vi "WriteWfmToDAQ.vi"(0 "clock settings":T3={"sample mode"=10178, "samples per channel"=1000, "rate"=1000.0} {"sample mode" items=["Finite Samples"=10178, "Continuous Samples"=10123, "Hardware Timed Single Point"=12522]}, 5 "channel settings":T2={"max value"=5.0, "min value"=-5.0, "physical channels"="Dev1/ai2", "input terminal configuration"=-1, "units"=10348} {"input terminal configuration" items=["Default"=-1, "RSE"=10083, "NRSE"=10078, "Differential"=10106, "Pseudodifferential"=12529]; "units" items=["Volts"=10348, "From Custom Scale"=10065]}, 9 "FuncGen settings":T1={"signal type"=enum."Sine Wave", "amplitude"=1.0, "frequency"=10.0, "noiseRMS"=1.0}, 11 "error in":errorcluster) -> (10 "error out":errorcluster)   [LabVIEW 2025]
uses:
  <vilib>/DAQmx/write.llb/DAQmx Write (Analog Wfm 1Chan NSamp).vi
  <vilib>/DAQmx/create/channels.llb/DAQmx Create Channel (AO-Voltage-Basic).vi
  <vilib>/DAQmx/configure/timing.llb/DAQmx Timing (Sample Clock).vi
  <vilib>/DAQmx/miscellaneous.llb/DAQmx Fill In Error Info.vi
  <resource>/objmgr/daqmx.rc
panel:
  out "Wfm":waveform(dbl)(graph)
  in  "stop":bool
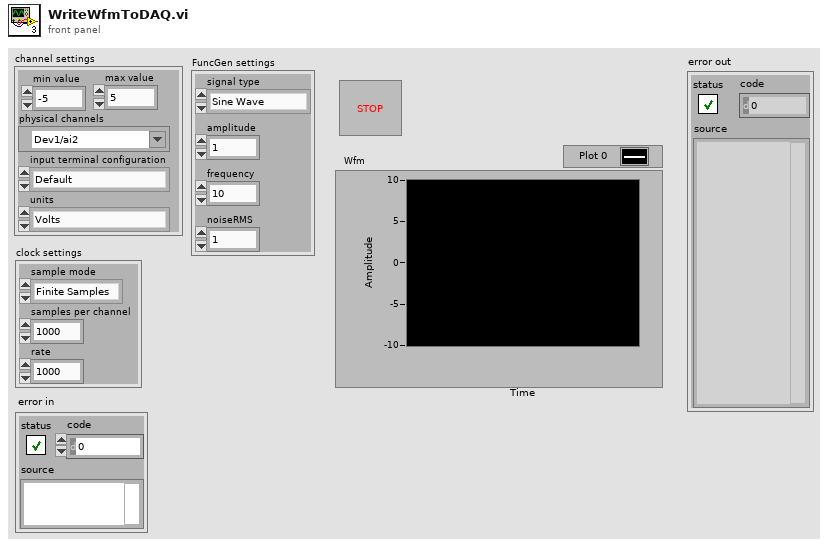
[diagram p1: front panel]
types:
  T1 = cluster{"signal type":enum16{"Sine Wave", "Triangle Wave", "Square Wave", "Sawtooth Wave"}, "amplitude":dbl, "frequency":dbl, "noiseRMS":dbl}
  T2 = cluster{"max value":dbl, "min value":dbl, "physical channels":tag, "input terminal configuration":i32, "units":i32}
  T3 = cluster{"sample mode":i32, "samples per channel":i32, "rate":dbl}
  T4 = enum16{"Sine Wave", "Triangle Wave", "Square Wave", "Sawtooth Wave"}
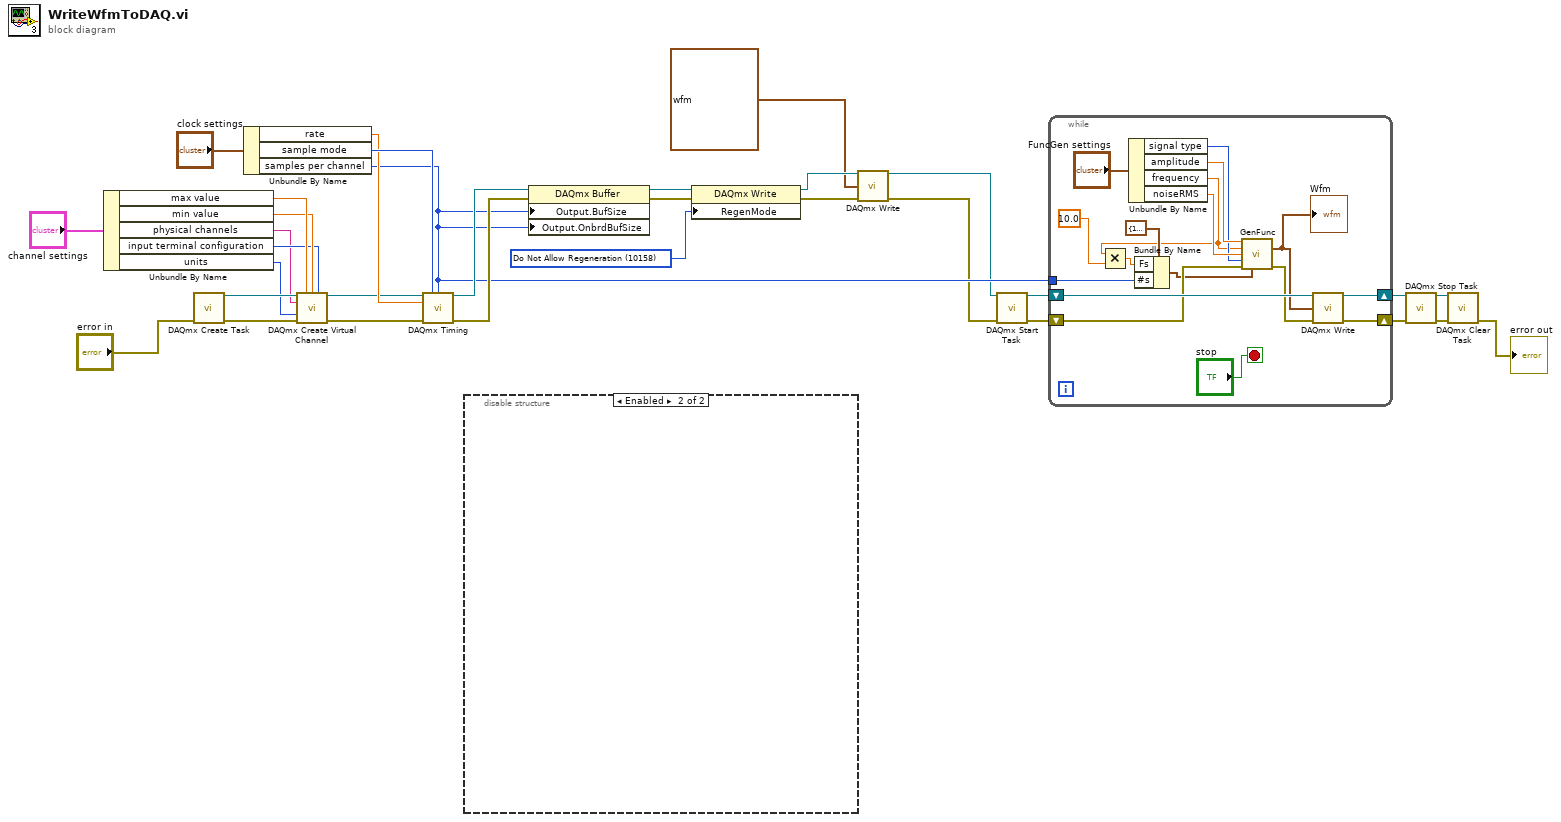
[diagram p0: block diagram]
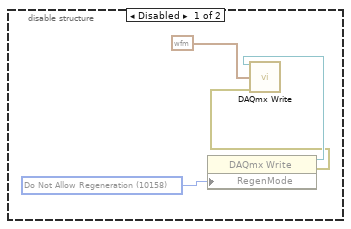
[diagram p2: hidden frame]
diagram:
  w8 = 10158 items=["Allow Regeneration"=10097, "Do Not Allow Regeneration"=10158] ("RegenMode")
  n1 = Unbundle By Name("channel settings") -> ("max value"=w27:dbl, "min value"=w26:dbl, "physical channels"=w24:tag, "input terminal configuration"=w25:i32, "units"=w23:i32)
  n2 = call <vilib>:"DAQmx Create Task.vi"("error in"="error in") -> ("task out"=w30:refnum<k21>, "error out"=w22:errorcluster)  [unwired: 13 in]
  n3 = Unbundle By Name("clock settings") -> ("rate"=w14:dbl, "sample mode"=w20:i32, "samples per channel"=w9:i32)
  n4 = call-poly <vilib>:"DAQmx Create Virtual Channel.vi"("task in"=w30, "maximum value"=w27, "minimum value"=w26, "output terminal configuration"=w25, "physical channels"=w24, "units"=w23, "error in"=w22) -> ("task out"=w13:refnum<k21>, "error out"=w12:errorcluster)  [unwired: 7 in]
  n5 = call-poly <vilib>:"DAQmx Timing.vi"("task/channels in"=w13, "sample mode"=w20, "samples per channel"=w9, "rate"=w14, "error in"=w12) -> ("task out"=w11:refnum<k21>, "error out"=w10:errorcluster)  [unwired: 9 in]
  n6 = disable-structure shown="Enabled" {
    frame Disabled {
      w38 = 10158 items=["Allow Regeneration"=10097, "Do Not Allow Regeneration"=10158] ("RegenMode")
      n7 = property class="DAQmx Write"("RegenMode"=w38) -> (reference=w36:refnum<k21>, reference out=w35:refnum<k21>, error in=w37:errorcluster, error out=w34:errorcluster)
      n8 = call-poly <vilib>:"DAQmx Write.vi"("task/channels in"=w35, "data"=waveform(dbl) {"t0"=timestamp(0 s since 1904-01-01), "dt"=0.0, "Y"=[]}, "error in"=w34) -> ("task out"=w40:refnum<k21>, "error out"=w39:errorcluster)  [unwired: 10 in, 1 out]
    }
    frame Enabled {
    }
  }
  n9 = property class="DAQmx Buffer"(reference=w11, error in=w10, "Output.BufSize"=w9, "Output.OnbrdBufSize"=w9) -> (reference out=w4:refnum<k21>, error out=w3:errorcluster)
  n10 = property class="DAQmx Write"(reference=w4, error in=w3, "RegenMode"=w8) -> (reference out=w7:refnum<k21>, error out=w6:errorcluster)
  n11 = call-poly <vilib>:"DAQmx Write.vi"("task/channels in"=w7, "data"=waveform(dbl) {"t0"=timestamp(0 s since 1904-01-01), "dt"=0.0, "Y"=[]}, "error in"=w6) -> ("task out"=w1:refnum<k21>, "error out"=w2:errorcluster)  [unwired: 10 in, 1 out]
  n12 = call <vilib>:"DAQmx Start Task.vi"("task/channels in"=w1, "error in"=w2) -> ("task out"=w18:refnum<k21>, "error out"=w15:errorcluster)  [unwired: 12 in]
  n13 = while {
    shift-right: [w51] -> w16
    shift-left: w18 -> [w53]
    shift-right: [w52] -> w17
    shift-left: w15 -> [w50]
    tunnel: w9 -> [w41]
    stop <- "stop" stop-if-true
    n14 = Unbundle By Name("FuncGen settings") -> ("signal type"=w54:T4, "amplitude"=w56:dbl, "frequency"=w43:dbl, "noiseRMS"=w55:dbl)
    n15 = Multiply(x=w43, y=10.0) -> (x*y=w44:dbl)
    n16 = Bundle By Name(cluster=cluster{"Fs":dbl, "#s":dbl} {"Fs"=1000.0, "#s"=1000.0} ("sampling info"), "Fs"=w44, "#s"=w41) -> (w46:cluster{"Fs":dbl, "#s":dbl})
    n17 = call "GenFunc.vi"("amplitude"=w56, "frequency"=w43, "noiseRMS"=w55, "signal type"=w54, "error in (no error)"=w50, "sampling info"=w46) -> ("signal out"=w47:waveform(dbl), "error out"=w49:errorcluster)  [unwired: 8 in]
    "Wfm" <- w47
    n18 = call-poly <vilib>:"DAQmx Write.vi"("task/channels in"=w53, "data"=w47, "error in"=w49) -> ("task out"=w51:refnum<k21>, "error out"=w52:errorcluster)  [unwired: 10 in, 1 out]
  }
  n19 = call <vilib>:"DAQmx Stop Task.vi"("task/channels in"=w16, "error in"=w17) -> ("task out"=w32:refnum<k21>, "error out"=w31:errorcluster)  [unwired: 12 in]
  n20 = call <vilib>:"DAQmx Clear Task.vi"("task in"=w32, "error in"=w31) -> ("error out"=→"error out":errorcluster)  [unwired: 13 in]
